vi "signalGenerator.vi"() -> ()   [LabVIEW 2024]
uses:
  <instrlib>/Rohde&Schwarz RF Signal Generator/Rohde&Schwarz RF Signal Generator.lvlib
panel:
  out "VISA resource name out":refnum<visa-resource-name>
  out "error out":errorcluster
  in  "Command":string
  in  "Digital Attenuation (0.0)":dbl format="%^.3e"
  in  "Offset (0.0)":dbl format="%^.3e"
  in  "Limit (30.0)":dbl=30.0 format="%^.3e"
  in  "Reset (T: Reset)":bool=TRUE
  out "VISA SG out":refnum<visa-resource-name>
  out "Error Out":errorcluster
  in  "Error In":errorcluster
  in  "START":bool
  in  "VISA signal generator":refnum<visa-resource-name>
  in  "RF Frequency (GHz)":dbl=44.0 min=0.0001 max=44.0
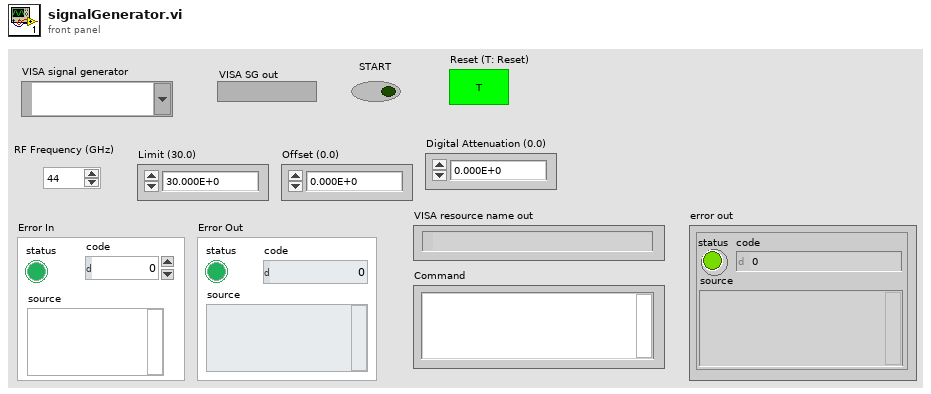
[diagram p1: front panel]
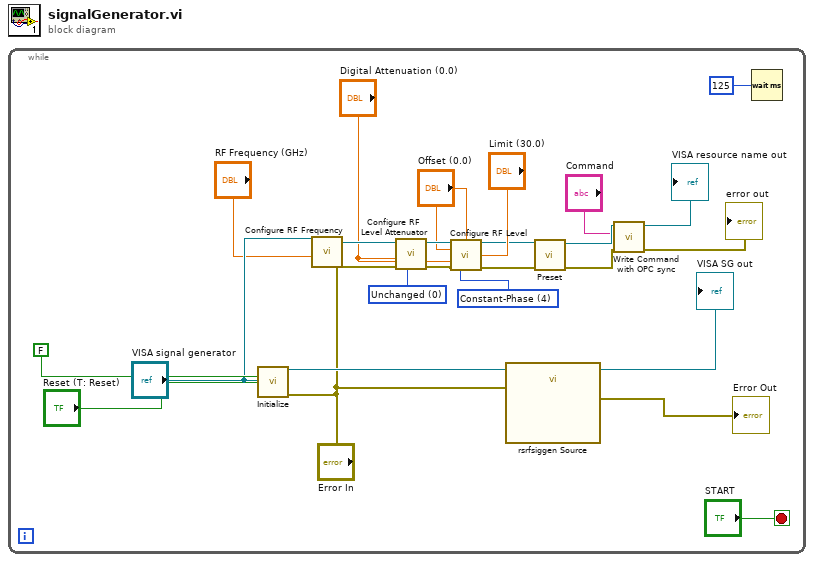
[diagram p0: block diagram]
diagram:
  n1 = while {
    stop <- "START" stop-if-true
    w12 = 4 items=["Auto", "Uninterrupted", "Strictly Monotone", "Constant-VSWR", "Constant-Phase"] ("Setting Characteristics (Constant-Phase)")
    w13 = 0 items=["Unchanged", "Full Attenuation"] ("RF OFF Mode (Unchanged)")
    n2 = call <instrlib>:"Initialize.vi"("VISA resource name"="VISA signal generator", "ID Query (T: Check)"=FALSE, "Reset (T: Reset)"="Reset (T: Reset)", "error in (no error)"="Error In") -> ("VISA resource name out"=w23:refnum<visa-resource-name>)  [unwired: 10 in, 1 out]
    n3 = call <instrlib>:"Configure RF Frequency.vi"("error in (no error)"="Error In", "Frequency (1GHz)"="RF Frequency (GHz)", "VISA resource name"="VISA signal generator") -> ("error out"=w17:errorcluster, "VISA resource name out"=w18:refnum<visa-resource-name>)  [unwired: 7 in]
    n4 = call <instrlib>:"Configure RF Level Attenuator.vi"("RF OFF Mode (Unchanged)"=w13, "error in (no error)"=w17, "Attenuation (0.0)"="Digital Attenuation (0.0)", "VISA resource name"=w18) -> ("error out"=w15:errorcluster, "VISA resource name out"=w16:refnum<visa-resource-name>)  [unwired: 6 in]
    n5 = call <instrlib>:"Configure RF Level.vi"("VISA resource name"=w16, "Offset (0.0)"="Offset (0.0)", "Path (1)"="Offset (0.0)", "Limit (30.0)"="Limit (30.0)", "Digital Attenuation (0.0)"="Digital Attenuation (0.0)", "error in (no error)"=w15, "Setting Characteristics (Constant-Phase)"=w12) -> ("VISA resource name out"=w11:refnum<visa-resource-name>, "error out"=w10:errorcluster)  [unwired: 7 in]
    n6 = call "rsrfsiggen Source.vi"("error in (no error)"="Error In", "instrument handle"=w23) -> ("error out"=→"Error Out":errorcluster, "instrument handle out"=→"VISA SG out":refnum<visa-resource-name>)  [unwired: 8 in]
    n7 = call <instrlib>:"Preset.vi"("error in (no error)"=w10, "VISA resource name"=w11) -> ("error out"=w7:errorcluster, "VISA resource name out"=w6:refnum<visa-resource-name>)  [unwired: 8 in]
    n8 = call <instrlib>:"Write Command with OPC sync.vi"("error in (no error)"=w7, "Command"="Command", "VISA resource name"=w6) -> ("error out"=→"error out":errorcluster, "VISA resource name out"=→"VISA resource name out":refnum<visa-resource-name>)  [unwired: 7 in]
    n9 = Wait (ms)(milliseconds to wait=u32 125 ("millisecond timer value")) -> ()  [unwired: 1 out]
  }
